vi "温升测试系统.vi"() -> ()   [LabVIEW 2021]
uses:
  <vilib>/Utility/NIReport.llb/Report Type.ctl
  <vilib>/Utility/file.llb/Write Delimited Spreadsheet (string).vi
  <vilib>/Utility/file.llb/Read Delimited Spreadsheet (string).vi
  <userlib>/_MGI/Timing/MGI Wait/MGI Wait (U32).vi
  <vilib>/Waveform/WDTFileIO.llb/Export Waveforms To Spreadsheet File (1D).vi
  <vilib>/Utility/NIReport.llb/Append Text Table to Report (wrap).vi
  <vilib>/Utility/NIReport.llb/NI_report.lvclass
  <vilib>/Utility/NIReport.llb/NI_ReportGenerationCore.lvlib
  <instrlib>/Keithley 27XX/Keithley 27XX.lvlib
  <vilib>/Utility/NIReport.llb/Excel/NI_Excel.lvclass
panel:
  in  "确定按钮 3":bool
  out "当前运行时间":dbl
  out "?":dbl
  in  "样品名称":string
  in  "文本下拉列表":u16(ring) items=["101", "102", "203"]
  out "?":dbl(slide) scale=0.0..200.0
  out "滑动杆":u8(slide) scale=0.0..100.0
  in  "确定按钮 2":bool
  in  "取消按钮":bool
  in  "首选项按钮":bool
  in  "保存按钮":bool
  in  "确定按钮":bool
  in  "停止按钮":bool
  in  "打开按钮":bool
  in  "新建按钮":bool
  in  "?":enum32{"温升曲线", "温升数据", "单曲线显示", "配置面板"}(tab)
  out "?":waveform(dbl)[](graph)
  out "?":i32(listbox)
  out "?":waveform(dbl)(graph)
  out "配置地址":i32(listbox)
  # "工况1"
  # "工况2"
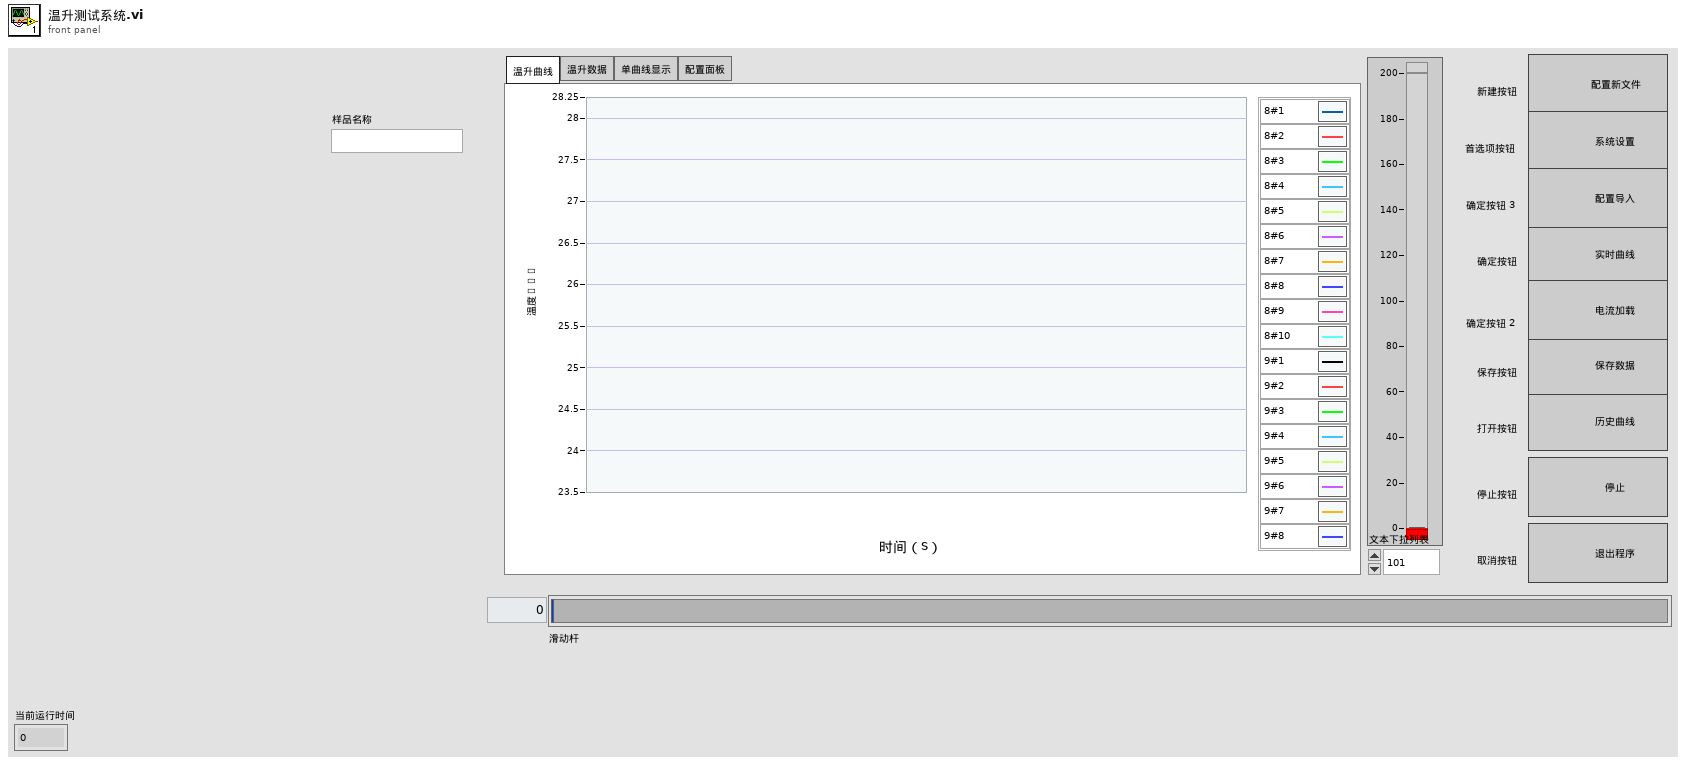
[diagram p1: front panel]
types:
  T1 = enum32{"Invalid", "Standard", "Closed", "Hidden", "Minimized", "Maximized"}
  T2 = cluster{"工况切换地址":refnum<visa-resource-name>, "温度读取":refnum<visa-resource-name>, "电流加载地址":refnum<visa-resource-name>, "RingText.Text":string, "工况1循环次数":dbl, "RingText.Text":string, "工况2循环次数":dbl, "大循环次数":dbl, "测试总时间":dbl, "扫描时间":dbl, "工况模式":enum16{"工况电流", "复合工况"}, "RingText.Text":string, "路径输出":path}
  T3 = typedef "NI_ReportGenerationCore.lvlib/Report Type.ctl" = enum16{"HTML", "Word", "Excel"}
  T4 = cluster{"all rows[0]":string, "all rows[1]":string, "all rows[2]":string, "all rows[3]":string, "all rows[4]":string, "all rows[5]":string, "all rows[6]":string, "all rows[7]":string, "all rows[8]":string, "all rows[9]":string, "all rows[10]":string, "all rows[11]":string, "all rows[12]":string}
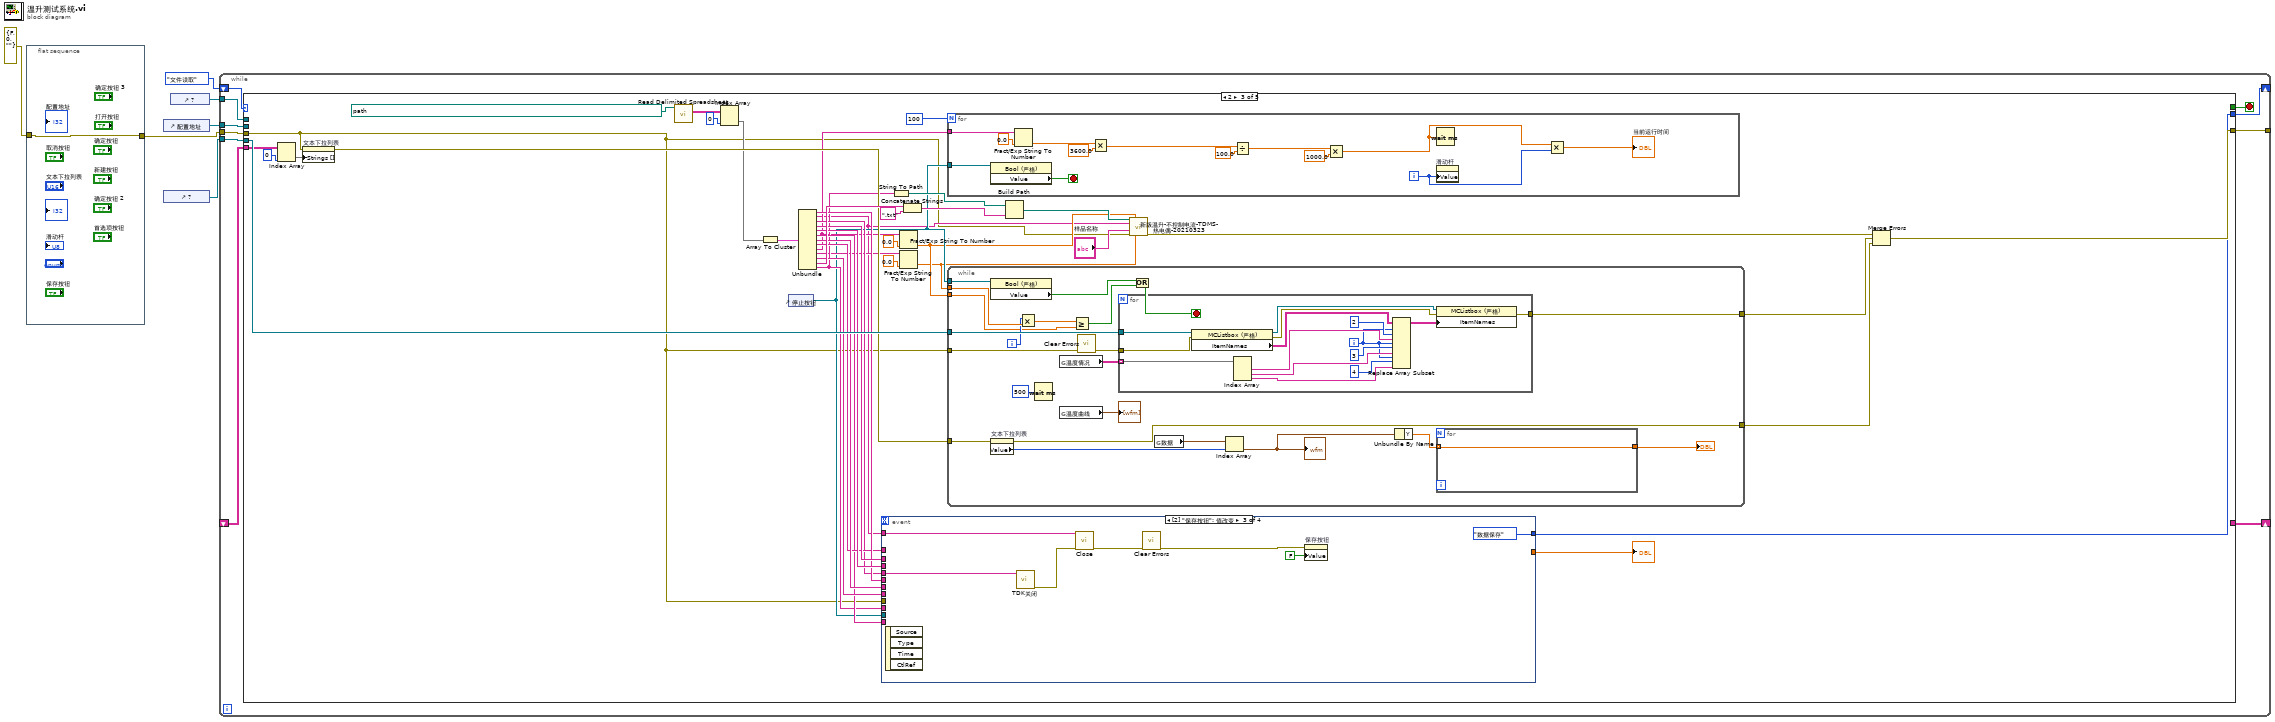
[diagram p0: block diagram]
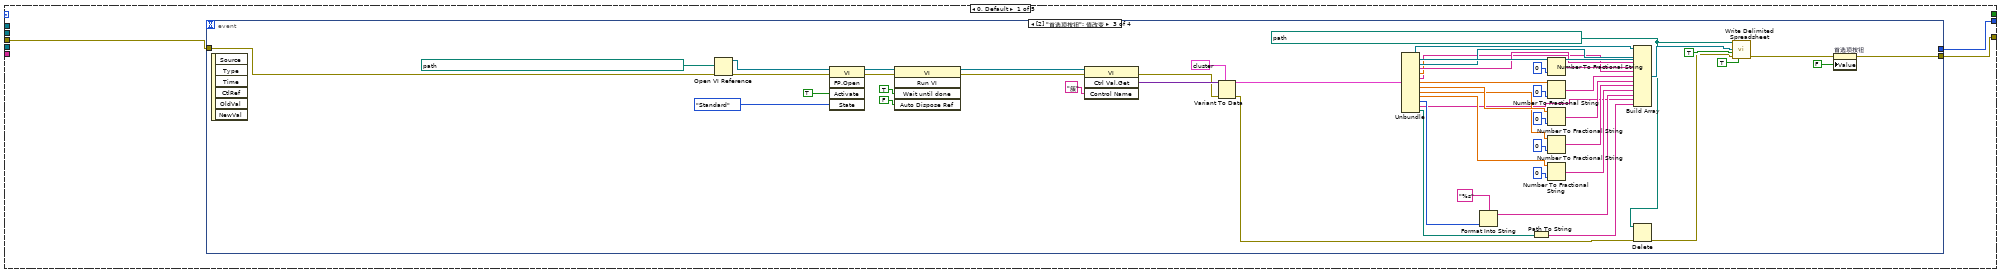
[diagram p2: hidden frame]
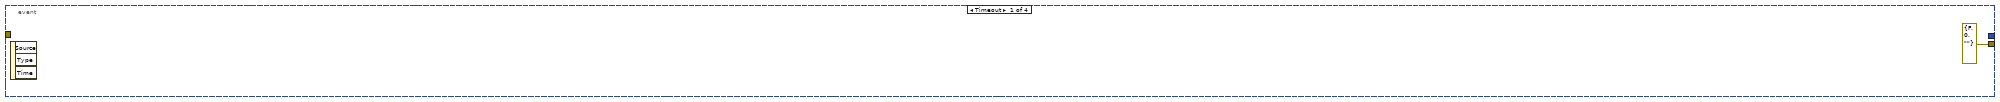
[diagram p3: hidden frame]
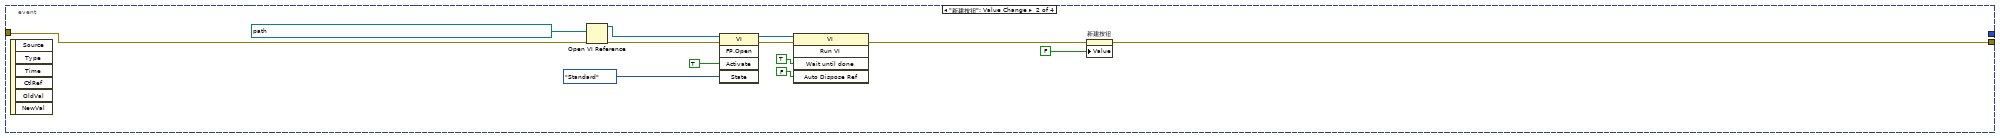
[diagram p4: hidden frame]
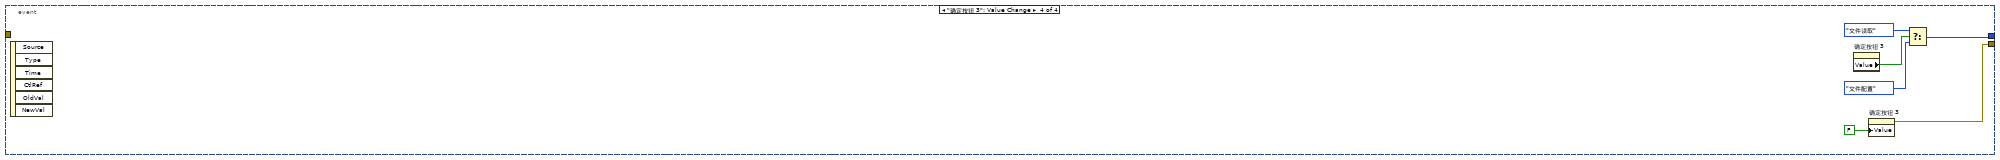
[diagram p5: hidden frame]
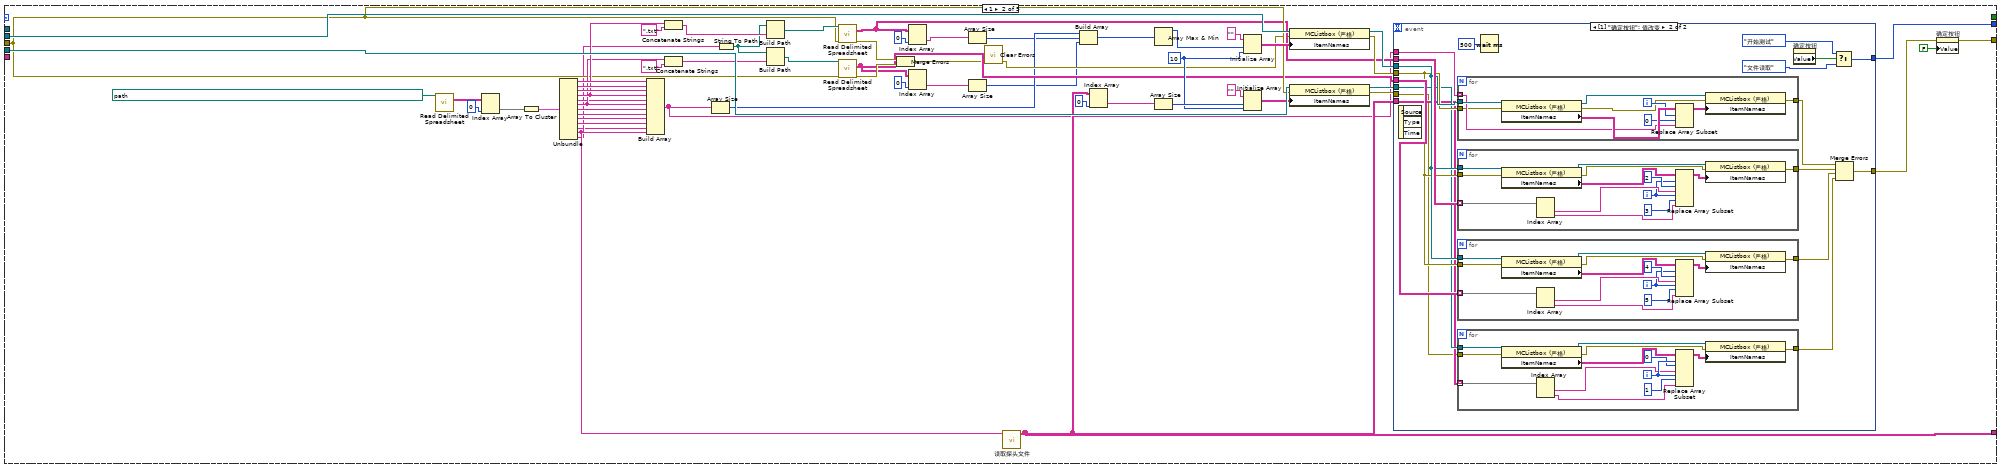
[diagram p6: hidden frame]
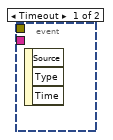
[diagram p7: hidden frame]
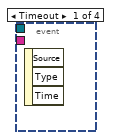
[diagram p8: hidden frame]
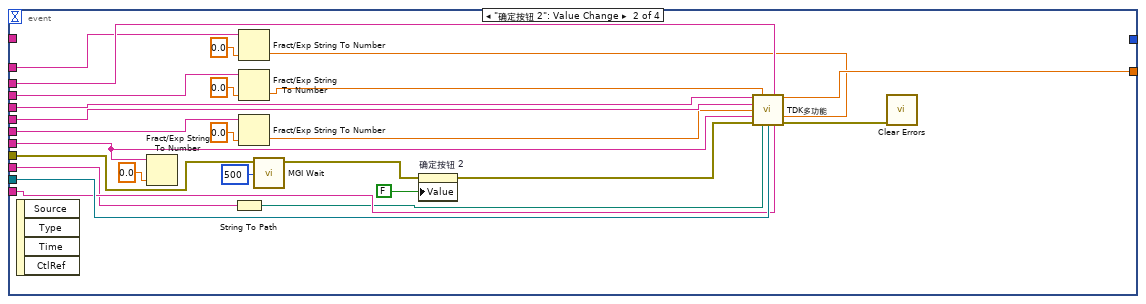
[diagram p9: hidden frame]
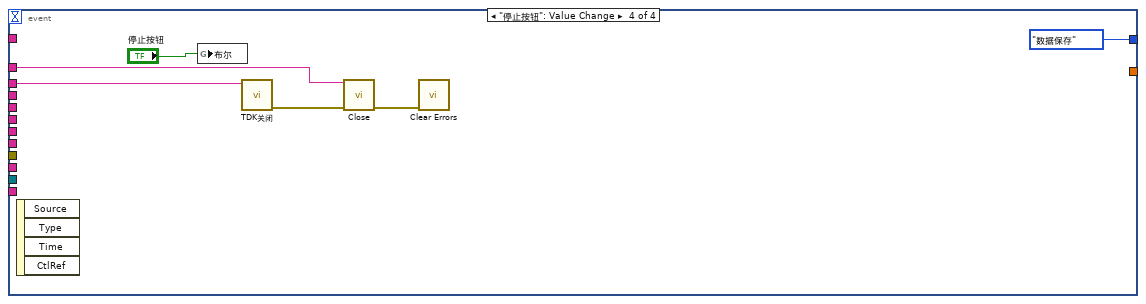
[diagram p10: hidden frame]
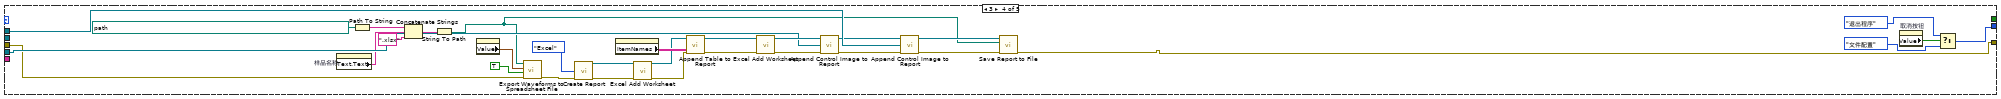
[diagram p11: hidden frame]
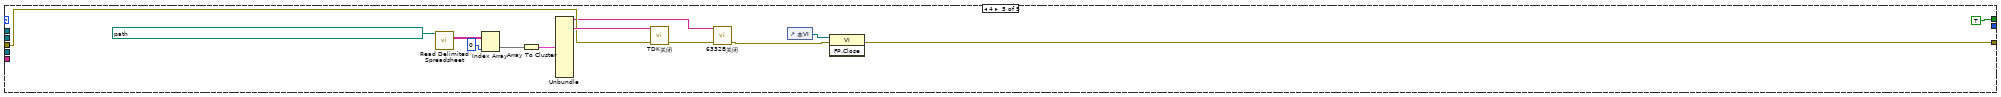
[diagram p12: hidden frame]
diagram:
  n1 = flat-sequence {
    tunnel: [w7] -> w2
    tunnel: errorcluster {"status"=FALSE, "code"=0, "source"=""} ("error in (no error)") -> [w7]
    frame #0 {
    }
  }
  n2 = control-ref of="配置地址"() -> (w5:refnum<vi>)
  n3 = control-ref of="?"() -> (w4:refnum<vi>)
  n4 = control-ref of="?"() -> (w3:refnum<vi>)
  n5 = while {
    tunnel: w5 -> [w17]
    tunnel: w4 -> [w16]
    shift-right: [w15] -> _
    shift-left: enum16{"文件读取", "文件配置", "开始测试", "数据保存", "退出程序"}."文件读取" -> [w8]
    shift-right: [w12] -> _
    shift-left: _ -> [w11]
    tunnel: w3 -> [w10]
    tunnel: w2 -> [w14]
    tunnel: [w13] -> _
    stop <- w9 stop-if-true
    n6 = case shown="2" w8 {
      tunnel: w17 -> [_ w153 _ _ _]
      tunnel: w16 -> [_ w152 w258 w367 _]
      tunnel: [w18 w93 w229 w356 _] -> w15
      tunnel: w14 -> [w19 w126 w223 w363 w393]
      tunnel: [w20 w95 w243 w352 w382] -> w13
      tunnel: [_ w119 _ _ _] -> w12
      tunnel: w11 -> [_ _ w257 _ _]
      tunnel: w10 -> [_ _ _ w366 _]
      tunnel: [_ _ _ _ TRUE] -> w9
      frame 0, Default {
        n7 = event shown="[2] \"首选项按钮\": 值改变" {
          selector: _ -> [_ _ _ _]
          dyn-events: _ -> [_ _ _ _]
          timeout: _ -> [_ _ _ _]
          tunnel: [errorcluster {"status"=FALSE, "code"=0, "source"=""} ("错误输出") w23 w36 w88] -> w20
          tunnel: w19 -> [_ w22 w35 _]
          tunnel: [_ _ _ w89] -> w18
          event Timeout {
            n8 = event-data() -> ()  [unwired: 1 in, 3 out]
          }
          event "新建按钮": Value Change {
            n9 = event-data() -> ()  [unwired: 1 in, 6 out]
            n10 = Open VI Reference(vi path=path "C:/Users/Administrator.CH-202202160008/Desktop/温升测试系统/文件写入.vi" ("VI路径"), error in (no error)=w22) -> (vi reference=w34:refnum<vi>, error out=w30:errorcluster)  [unwired: 4 in]
            n11 = invoke class="VI" method="FP.Open"(reference=w34, error in=w30, "Activate"=TRUE ("激活？"), "State"=T1."Standard" ("状态")) -> (reference out=w33:refnum<vi>, error out=w29:errorcluster)  [unwired: 1 in, 3 out]
            n12 = invoke class="VI" method="Run VI"(reference=w33, error in=w29, "Wait until done"=TRUE ("结束前等待"), "Auto Dispose Ref"=FALSE ("自动销毁引用")) -> (error out=w25:errorcluster)  [unwired: 1 in, 4 out]
            n13 = property on="新建按钮" class="Bool (严格)"(error in=w25, "Value"=FALSE ("新建按钮")) -> (error out=w23:errorcluster)  [unwired: 1 in, 1 out]
          }
          event "首选项按钮": Value Change {
            w37 = path "C:/Users/Administrator.CH-202202160008/Desktop/温升测试系统/仪器配置文件/仪器配置.txt" ("file path (dialog if empty)")
            n14 = event-data() -> ()  [unwired: 1 in, 6 out]
            n15 = Open VI Reference(vi path=path "C:/Users/Administrator.CH-202202160008/Desktop/温升测试系统/系统设置.vi" ("VI路径"), error in (no error)=w35) -> (vi reference=w86:refnum<vi>, error out=w82:errorcluster)  [unwired: 4 in]
            n16 = invoke class="VI" method="FP.Open"(reference=w86, error in=w82, "Activate"=TRUE ("激活？"), "State"=T1."Standard" ("状态")) -> (reference out=w85:refnum<vi>, error out=w81:errorcluster)  [unwired: 1 in, 3 out]
            n17 = invoke class="VI" method="Run VI"(reference=w85, error in=w81, "Wait until done"=TRUE ("结束前等待"), "Auto Dispose Ref"=FALSE ("自动销毁引用")) -> (reference out=w74:refnum<vi>, error out=w73:errorcluster)  [unwired: 1 in, 3 out]
            n18 = invoke class="VI" method="Ctrl Val.Get"(reference=w74, error in=w73, "Control Name"="簇" ("控件名")) -> (error out=w72:errorcluster, "Get Control Value Variant"=w77:variant)  [unwired: 1 in, 2 out]
            n19 = Variant To Data(error in=w72, type=T2 {"工况切换地址"="", "温度读取"="", "电流加载地址"="", "RingText.Text"="新建 文本文档", "工况1循环次数"=1.0, "RingText.Text"="±300", "工况2循环次数"=1.0, "大循环次数"=1.0, "测试总时间"=53.0, "扫描时间"=53.0, "工况模式"=enum."复合工况", "RingText.Text"="", "路径输出"=path "C:/Users/Administrator.CH-202202160008/Desktop/温升测试系统/温升配置文件"} ("簇"), Variant=w77) -> (data=w70:T2, error out=w40:errorcluster)
            n20 = Unbundle(w70) -> ("工况切换地址"=w69:refnum<visa-resource-name>, "温度读取"=w68:refnum<visa-resource-name>, "电流加载地址"=w67:refnum<visa-resource-name>, "RingText.Text"=w66:string, "工况1循环次数"=w65:dbl, "RingText.Text"=w58:string, "工况2循环次数"=w57:dbl, "大循环次数"=w55:dbl, "测试总时间"=w53:dbl, "扫描时间"=w51:dbl, "工况模式"=w49:enum16{"工况电流", "复合工况"}, "RingText.Text"=w46:string, "路径输出"=w45:path)
            n21 = Format Into String(format string="%s" ("格式字符串"), w49) -> (resulting string=w47:string)  [unwired: 2 in, 1 out]
            n22 = Path To String(path=w45) -> (string=w44:string)
            n23 = Number To Fractional String(number=w65, precision (6)=i16 0 ("精度(6)")) -> (F-format string=w64:string)  [unwired: 2 in]
            n24 = Number To Fractional String(number=w57, precision (6)=i16 0 ("精度(6)")) -> (F-format string=w56:string)  [unwired: 2 in]
            n25 = Number To Fractional String(number=w55, precision (6)=i16 0 ("精度(6)")) -> (F-format string=w54:string)  [unwired: 2 in]
            n26 = Number To Fractional String(number=w53, precision (6)=i16 0 ("精度(6)")) -> (F-format string=w52:string)  [unwired: 2 in]
            n27 = Number To Fractional String(number=w51, precision (6)=i16 0 ("精度(6)")) -> (F-format string=w50:string)  [unwired: 2 in]
            n28 = Build Array(w69, w68, w67, w66, w64, w58, w56, w54, w52, w50, w47, w46, w44) -> (w43:refnum<visa-resource-name>[])
            n29 = Delete(path (use dialog)=w37, error in=w40) -> (error out=w39:errorcluster)  [unwired: 3 in, 2 out]
            n30 = call-poly <vilib>:"Write Delimited Spreadsheet.vi"("file path (dialog if empty)"=w37, "1D data"=w43, "append to file? (new file:F)"=TRUE, "error in (no error)"=w39, "transpose? (no:F)"=TRUE) -> ("error out"=w38:errorcluster)  [unwired: 9 in, 1 out]
            n31 = property on="首选项按钮" class="Bool (严格)"(error in=w38, "Value"=FALSE ("首选项按钮")) -> (error out=w36:errorcluster)  [unwired: 1 in, 1 out]
          }
          event "确定按钮 3": Value Change {
            n32 = event-data() -> ()  [unwired: 1 in, 6 out]
            n33 = property on="确定按钮 3" class="Bool (严格)"() -> ("Value"=w92:bool)  [unwired: 2 in, 2 out]
            n34 = property on="确定按钮 3" class="Bool (严格)"("Value"=FALSE ("确定按钮 3")) -> (error out=w88:errorcluster)  [unwired: 2 in, 1 out]
            n35 = Select(t=enum16{"文件配置", "文件读取", "开始测试", "数据保存", "退出程序"}."文件读取", s=w92, f=enum16{"文件配置", "文件读取", "开始测试", "数据保存", "退出程序"}."文件配置") -> (s? t:f=w89:enum16{"文件配置", "文件读取", "开始测试", "数据保存", "退出程序"})
          }
        }
      }
      frame 1 {
        w137 = 10 ("维数大小")
        n36 = call-poly <vilib>:"Read Delimited Spreadsheet.vi"("file path (dialog if empty)"=path "C:/Users/Administrator.CH-202202160008/Desktop/温升测试系统/仪器配置文件/仪器配置.txt") -> ("all rows"=w117:string[][])  [unwired: 9 in, 5 out]
        n37 = Index Array(array=w117, index (col)=0 ("禁用的索引 (列)")) -> (element=w115:string[])  [unwired: 1 in]
        n38 = Array To Cluster(array=w115) -> (cluster=w114:T4)
        n39 = Unbundle(w114) -> ("all rows[0]"=w147:string, "all rows[1]"=w146:string, "all rows[2]"=w145:string, "all rows[3]"=w140:string, "all rows[4]"=w113:string, "all rows[5]"=w132:string, "all rows[6]"=w112:string, "all rows[7]"=w111:string, "all rows[8]"=w110:string, "all rows[9]"=w109:string, "all rows[10]"=w106:string, "all rows[11]"=w144:string, "all rows[12]"=w108:string)
        n40 = Build Array(w147, w146, w145, w140, w113, w132, w112, w111, w110, w109, w106, w144) -> (w103:string[])
        n41 = Concatenate Strings(w140, ".txt" ("字符串")) -> (w141:string)
        n42 = Concatenate Strings(w132, ".txt" ("字符串")) -> (w133:string)
        n43 = Array Size(array=w103) -> (size(s)=w102:i32)
        n44 = String To Path(string=w108) -> (path=w107:path)
        n45 = Build Path(base path=w107, name or relative path=w141) -> (appended path=w143:path)
        n46 = Build Path(base path=w107, name or relative path=w133) -> (appended path=w130:path)
        n47 = call-poly <vilib>:"Read Delimited Spreadsheet.vi"("file path (dialog if empty)"=w143, "error in (no error)"=w126) -> ("all rows"=w122:string[][], "error out"=w128:errorcluster)  [unwired: 8 in, 4 out]
        n48 = call-poly <vilib>:"Read Delimited Spreadsheet.vi"("file path (dialog if empty)"=w130, "error in (no error)"=w126) -> ("all rows"=w124:string[][], "error out"=w127:errorcluster)  [unwired: 8 in, 4 out]
        n49 = Merge Errors(w128, w127) -> (w104:errorcluster)
        n50 = Index Array(array=w122, index (col)=0 ("禁用的索引 (列)")) -> (element=w136:string[])  [unwired: 1 in]
        n51 = Index Array(array=w124, index (col)=0 ("禁用的索引 (列)")) -> (element=w129:string[])  [unwired: 1 in]
        n52 = Array Size(array=w136) -> (size(s)=w101:i32)
        n53 = Array Size(array=w129) -> (size(s)=w100:i32)
        n54 = call <vilib>:"Clear Errors.vi"("error in (no error)"=w104) -> ("error out"=w105:errorcluster)  [unwired: 5 in, 1 out]
        n55 = call "读取探头文件.vi"("字符串"=w144) -> ("all rows"=w119:string[][])  [unwired: 10 in]
        n56 = Build Array(w102, w101, w100) -> (w99:i32[])
        n57 = Index Array(array=w119, index (col)=0 ("禁用的索引 (列)")) -> (element=w148:string[])  [unwired: 1 in]
        n58 = Array Size(array=w148) -> (size(s)=w149:i32)
        n59 = Array Max & Min(array=w99) -> (max value=w98:i32)  [unwired: 3 out]
        n60 = Initialize Array("" ("元素"), w98, w137) -> (w139:string[][])
        n61 = Initialize Array("", w149, w137) -> (w150:string[][])
        n62 = property class="MCListbox (严格)"(reference=w153, error in=w105, "ItemNames"=w139) -> (reference out=w125:refnum<vi>, error out=w123:errorcluster)
        n63 = property class="MCListbox (严格)"(reference=w152, error in=w126, "ItemNames"=w150) -> (reference out=w121:refnum<vi>, error out=w120:errorcluster)
        n64 = event shown="[1] \"确定按钮\": 值改变" {
          selector: _ -> [_ _]
          dyn-events: _ -> [_ _]
          timeout: _ -> [_ _]
          tunnel: w125 -> [_ w165]
          tunnel: w124 -> [_ w167]
          tunnel: w123 -> [_ w163]
          tunnel: w122 -> [_ w166]
          tunnel: w103 -> [_ w164]
          tunnel: w121 -> [_ w162]
          tunnel: w119 -> [_ w161]
          tunnel: w120 -> [_ w160]
          tunnel: [_ w159] -> w96
          tunnel: [_ w154] -> w93
          event Timeout {
            n65 = event-data() -> ()  [unwired: 1 in, 3 out]
          }
          event "确定按钮": Value Change {
            n66 = event-data() -> ()  [unwired: 1 in, 3 out]
            n67 = for {
              tunnel: w165 -> [w207]
              tunnel: w164 -> [w202] mode=indexing
              tunnel: w163 -> [w201]
              tunnel: [w200] -> w168
              i -> [w204]
              n68 = property class="MCListbox (严格)"(reference=w207, error in=w201) -> (reference out=w199:refnum<vi>, error out=w198:errorcluster, "ItemNames"=w206:string[][])
              n69 = Replace Array Subset(array=w206, new element=w202, index (row)=w204, index (col)=0 ("禁用的索引 (列)")) -> (w205:string[][])
              n70 = property class="MCListbox (严格)"(reference=w199, error in=w198, "ItemNames"=w205) -> (error out=w200:errorcluster)  [unwired: 1 out]
            }
            n71 = for {
              tunnel: w165 -> [w197]
              tunnel: w166 -> [w193] mode=indexing
              tunnel: w163 -> [w188]
              tunnel: [w187] -> w169
              i -> [w190]
              n72 = property class="MCListbox (严格)"(reference=w197, error in=w188) -> (reference out=w186:refnum<vi>, error out=w185:errorcluster, "ItemNames"=w196:string[][])
              n73 = Index Array(array=w193) -> (element #1=w192:string, element #2=w191:string)  [unwired: 2 in]
              n74 = Replace Array Subset(array=w196, new element #1=w192, index (row) #1=w190, index (col) #1=2 ("禁用的索引 (列)"), new element #2=w191, index (row) #2=w190, index (col) #2=3 ("禁用的索引 (列)")) -> (w195:string[][])
              n75 = property class="MCListbox (严格)"(reference=w186, error in=w185, "ItemNames"=w195) -> (error out=w187:errorcluster)  [unwired: 1 out]
            }
            n76 = for {
              tunnel: w165 -> [w184]
              tunnel: w167 -> [w176] mode=indexing
              tunnel: w163 -> [w173]
              tunnel: [w172] -> w170
              i -> [w178]
              n77 = property class="MCListbox (严格)"(reference=w184, error in=w173) -> (reference out=w175:refnum<vi>, error out=w174:errorcluster, "ItemNames"=w183:string[][])
              n78 = Index Array(array=w176) -> (element #1=w180:string, element #2=w179:string)  [unwired: 2 in]
              n79 = Replace Array Subset(array=w183, new element #1=w180, index (row) #1=w178, index (col) #1=4 ("禁用的索引 (列)"), new element #2=w179, index (row) #2=w178, index (col) #2=5 ("禁用的索引 (列)")) -> (w182:string[][])
              n80 = property class="MCListbox (严格)"(reference=w175, error in=w174, "ItemNames"=w182) -> (error out=w172:errorcluster)  [unwired: 1 out]
            }
            n81 = for {
              tunnel: w162 -> [w220]
              tunnel: w161 -> [w214] mode=indexing
              tunnel: w160 -> [w209]
              tunnel: [w208] -> w171
              i -> [w217]
              n82 = property class="MCListbox (严格)"(reference=w220, error in=w209) -> (reference out=w211:refnum<vi>, error out=w210:errorcluster, "ItemNames"=w219:string[][])
              n83 = Index Array(array=w214) -> (element #1=w213:string, element #2=w212:string)  [unwired: 2 in]
              n84 = Replace Array Subset(array=w219, new element #1=w213, index (row) #1=w217, index (col) #1=0 ("禁用的索引 (列)"), new element #2=w212, index (row) #2=w217, index (col) #2=1 ("禁用的索引 (列)")) -> (w218:string[][])
              n85 = property class="MCListbox (严格)"(reference=w211, error in=w210, "ItemNames"=w218) -> (error out=w208:errorcluster)  [unwired: 1 out]
            }
            n86 = Wait (ms)(milliseconds to wait=u32 500 ("等待时间（毫秒）")) -> ()  [unwired: 1 out]
            n87 = property on="确定按钮" class="Bool (严格)"() -> ("Value"=w157:bool)  [unwired: 2 in, 2 out]
            n88 = Select(t=enum16{"文件配置", "文件读取", "开始测试", "数据保存", "退出程序"}."开始测试", s=w157, f=enum16{"文件配置", "文件读取", "开始测试", "数据保存", "退出程序"}."文件读取") -> (s? t:f=w154:enum16{"文件配置", "文件读取", "开始测试", "数据保存", "退出程序"})
            n89 = Merge Errors(w168, w169, w170, w171) -> (w159:errorcluster)
          }
        }
        n90 = property on="确定按钮" class="Bool (严格)"(error in=w96, "Value"=FALSE ("确定按钮")) -> (error out=w95:errorcluster)  [unwired: 1 in, 1 out]
      }
      frame 2 {
        n91 = Index Array(array=w257, index (col)=0 ("禁用的索引 (列)")) -> (element=w255:string[])  [unwired: 1 in]
        n92 = property on="文本下拉列表" class="Ring (严格)"(error in=w223, "Strings []"=w255) -> (error out=w246:errorcluster)  [unwired: 1 in, 1 out]
        n93 = call-poly <vilib>:"Read Delimited Spreadsheet.vi"("file path (dialog if empty)"=path "C:/Users/Administrator.CH-202202160008/Desktop/温升测试系统/仪器配置文件/仪器配置.txt") -> ("all rows"=w239:string[][])  [unwired: 9 in, 5 out]
        n94 = Index Array(array=w239, index (col)=0 ("禁用的索引 (列)")) -> (element=w237:string[])  [unwired: 1 in]
        n95 = Array To Cluster(array=w237) -> (cluster=w236:T4)
        n96 = control-ref of="停止按钮"() -> (w228:refnum<vi>)
        n97 = Unbundle(w236) -> ("all rows[0]"=w252:string, "all rows[1]"=w225:string, "all rows[2]"=w241:string, "all rows[3]"=w253:string, "all rows[4]"=w254:string, "all rows[5]"=w248:string, "all rows[6]"=w251:string, "all rows[7]"=w249:string, "all rows[8]"=w231:string, "all rows[9]"=w230:string, "all rows[10]"=w250:string, "all rows[11]"=w260:string, "all rows[12]"=w233:string)
        n98 = event shown="[2] \"保存按钮\": 值改变" {
          selector: _ -> [_ _ _ _]
          dyn-events: _ -> [_ _ _ _]
          timeout: _ -> [_ _ _ _]
          tunnel: w241 -> [_ w337 w344 _]
          tunnel: w254 -> [_ w327 _ _]
          tunnel: w253 -> [_ w336 _ w347]
          tunnel: w252 -> [_ w335 _ _]
          tunnel: w251 -> [_ w325 _ _]
          tunnel: w250 -> [_ w319 _ _]
          tunnel: w249 -> [_ w323 _ w346]
          tunnel: w223 -> [_ w317 _ _]
          tunnel: w233 -> [_ w321 _ _]
          tunnel: w228 -> [_ w334 _ _]
          tunnel: w248 -> [_ w333 _ _]
          tunnel: [_ w332 _ _] -> w247
          tunnel: [_ _ enum16{"文件配置", "文件读取", "开始测试", "数据保存", "退出程序"}."数据保存" enum16{"文件配置", "文件读取", "开始测试", "数据保存", "退出程序"}."数据保存"] -> w229
          tunnel: w225 -> [_ _ w342 _]
          event Timeout {
            n99 = event-data() -> ()  [unwired: 1 in, 3 out]
          }
          event "确定按钮 2": Value Change {
            n100 = event-data() -> ()  [unwired: 1 in, 4 out]
            n101 = Fract/Exp String To Number(string=w319, default (0 dbl)=0.0 ("默认(0 DBL)")) -> ()  [unwired: 2 in, 2 out]
            n102 = String To Path(string=w321) -> (path=w320:path)
            n103 = Fract/Exp String To Number(string=w323, default (0 dbl)=0.0 ("默认(0 DBL)")) -> (number=w322:dbl)  [unwired: 2 in, 1 out]
            n104 = Fract/Exp String To Number(string=w327, default (0 dbl)=0.0 ("默认(0 DBL)")) -> (number=w326:dbl)  [unwired: 2 in, 1 out]
            n105 = Fract/Exp String To Number(string=w325, default (0 dbl)=0.0 ("默认(0 DBL)")) -> (number=w324:dbl)  [unwired: 2 in, 1 out]
            n106 = call-poly <userlib>:"MGI Wait.vi"("ms"=u32 500, "Error In"=w317) -> ("Error Out"=w315:errorcluster)  [unwired: 5 in]
            n107 = property on="确定按钮 2" class="Bool (严格)"(error in=w315, "Value"=FALSE ("确定按钮 2")) -> (error out=w314:errorcluster)  [unwired: 1 in, 1 out]
            n108 = call "TDK多功能.vi"("TDK地址"=w337, "工况1循环次数"=w326, "工况1"=w336, "工况切换地址"=w335, "工况2循环次数"=w324, "字符串"=w319, "大循环次数"=w322, "错误输入（无错误）"=w314, "工况地址"=w320, "Bool引用句柄"=w334, "工况2"=w333) -> ("运行总时间"=w332:dbl, "错误输出"=w313:errorcluster)  [unwired: 3 in]
            n109 = call <vilib>:"Clear Errors.vi"("error in (no error)"=w313) -> ()  [unwired: 5 in, 2 out]
          }
          event "保存按钮": Value Change {
            n110 = event-data() -> ()  [unwired: 1 in, 4 out]
            n111 = call "TDK关闭.vi"("VISA resource name"=w344) -> ("error out"=w341:errorcluster)  [unwired: 10 in]
            n112 = call <instrlib>:"Close.vi"("VISA resource name"=w342, "error in (no error)"=w341) -> ("error out"=w339:errorcluster)  [unwired: 13 in]
            n113 = call <vilib>:"Clear Errors.vi"("error in (no error)"=w339) -> ("error out"=w338:errorcluster)  [unwired: 5 in, 1 out]
            n114 = property on="保存按钮" class="Bool (严格)"(error in=w338, "Value"=FALSE ("保存按钮")) -> ()  [unwired: 1 in, 2 out]
          }
          event "停止按钮": Value Change {
            n115 = event-data() -> ()  [unwired: 1 in, 4 out]
            n116 = global write "数据传输.vi" "布尔"("停止按钮") -> ()
            n117 = call "TDK关闭.vi"("VISA resource name"=w347) -> ("error out"=w350:errorcluster)  [unwired: 10 in]
            n118 = call <instrlib>:"Close.vi"("VISA resource name"=w346, "error in (no error)"=w350) -> ("error out"=w349:errorcluster)  [unwired: 13 in]
            n119 = call <vilib>:"Clear Errors.vi"("error in (no error)"=w349) -> ()  [unwired: 5 in, 2 out]
          }
        }
        "?" <- w247
        n120 = String To Path(string=w233) -> (path=w232:path)
        n121 = Fract/Exp String To Number(string=w231, default (0 dbl)=0.0 ("默认(0 DBL)")) -> (number=w226:dbl)  [unwired: 2 in, 1 out]
        n122 = Fract/Exp String To Number(string=w230, default (0 dbl)=0.0 ("默认(0 DBL)")) -> (number=w222:dbl)  [unwired: 2 in, 1 out]
        n123 = Concatenate Strings(w260, ".txt" ("字符串")) -> (w259:string)
        n124 = for {
          N: 100 -> [_]
          tunnel: w231 -> [w306]
          tunnel: w228 -> [w304]
          i -> [w308]
          stop <- w303 stop-if-true
          n125 = property class="Bool (严格)"(reference=w304) -> ("Value"=w303:bool)  [unwired: 1 in, 2 out]
          n126 = Fract/Exp String To Number(string=w306, default (0 dbl)=0.0 ("默认(0 DBL)")) -> (number=w301:dbl)  [unwired: 2 in, 1 out]
          n127 = Multiply(x=w301, y=3600.0) -> (x*y=w300:dbl)
          n128 = Divide(x=w300, y=100.0) -> (x/y=w310:dbl)
          n129 = Multiply(x=w310, y=1000.0) -> (x*y=w309:dbl)
          n130 = Wait (ms)(milliseconds to wait=w309) -> ()  [unwired: 1 out]
          n131 = property on="滑动杆" class="Slide (严格)"("Value"=w308) -> ()  [unwired: 2 in, 2 out]
          n132 = Multiply(x=w309, y=w308) -> (x*y=→"当前运行时间":dbl)
        }
        n133 = while {
          tunnel: w258 -> [w283]
          tunnel: w246 -> [w282]
          tunnel: [w280] -> w244
          tunnel: w223 -> [w279]
          tunnel: [w281] -> w245
          tunnel: w222 -> [w272]
          tunnel: w226 -> [w269]
          tunnel: w228 -> [w268]
          i -> [w271]
          stop <- w265 stop-if-true
          n134 = property class="Bool (严格)"(reference=w268) -> ("Value"=w267:bool)  [unwired: 1 in, 2 out]
          n135 = property on="文本下拉列表" class="Ring (严格)"(error in=w282) -> (error out=w280:errorcluster, "Value"=w276:u16)  [unwired: 1 in, 1 out]
          n136 = Multiply(x=w271, y=w272) -> (x*y=w270:dbl)
          n137 = Wait (ms)(milliseconds to wait=u32 500 ("等待时间（毫秒）")) -> ()  [unwired: 1 out]
          n138 = global read "数据传输.vi" "温度情况"() -> (w264:string[][])
          n139 = global read "数据传输.vi" "温度曲线"() -> (→"?":waveform(dbl)[])
          n140 = Greater Or Equal?(x=w270, y=w269) -> (x >= y?=w266:bool)
          n141 = call <vilib>:"Clear Errors.vi"("error in (no error)"=w279) -> ("error out"=w278:errorcluster)  [unwired: 5 in, 1 out]
          n142 = for {
            tunnel: w283 -> [w299]
            tunnel: w264 -> [w294] mode=indexing
            tunnel: w278 -> [w289]
            tunnel: [w288] -> w281
            i -> [w287]
            n143 = property class="MCListbox (严格)"(reference=w299, error in=w289) -> (reference out=w291:refnum<vi>, error out=w290:errorcluster, "ItemNames"=w298:string[][])
            n144 = Index Array(array=w294) -> (element #1=w293:string, element #2=w292:string, element #3=w285:string)  [unwired: 3 in]
            n145 = Replace Array Subset(array=w298, new element #1=w293, index (row) #1=w287, index (col) #1=2 ("禁用的索引 (列)"), new element #2=w292, index (row) #2=w287, index (col) #2=3 ("禁用的索引 (列)"), new element #3=w285, index (row) #3=w287, index (col) #3=4 ("禁用的索引 (列)")) -> (w297:string[][])
            n146 = property class="MCListbox (严格)"(reference=w291, error in=w290, "ItemNames"=w297) -> (error out=w288:errorcluster)  [unwired: 1 out]
          }
          n147 = Or(x=w267, y=w266) -> (x .or. y?=w265:bool)
          n148 = global read "数据传输.vi" "数据"() -> (w262:waveform(dbl)[])
          n149 = Index Array(array=w262, index=w276) -> (element=w275:waveform(dbl))
          "?" <- w275
          n150 = Unbundle By Name(w275) -> ("Y"=w274:dbl[])
          n151 = for {
            tunnel: w274 -> [w284] mode=indexing
            tunnel: [w284] -> w273
          }
          "?" <- w273
        }
        n152 = Build Path(base path=w232, name or relative path=w259) -> (appended path=w227:path)
        n153 = call "新版温升-不控制电流-TDMS-热电偶-20210323.vi"("file path (dialog if empty)"=w227, "总记录时间（H）"=w226, "温度读取地址"=w225, "样品名称"="样品名称", "error in (no error)"=w223, "延迟时间（s）"=w222) -> ("错误输出"=w221:errorcluster)  [unwired: 4 in, 5 out]
        n154 = Merge Errors(w221, w245, w244) -> (w243:errorcluster)
      }
      frame 3 {
        n155 = property on="样品名称" class="Str"() -> ("Text.Text"=w362:string)  [unwired: 2 in, 2 out]
        n156 = Path To String(path=path "C:/Users/Administrator.CH-202202160008/Desktop/温升测试系统/实验数据" ("report file path")) -> (string=w359:string)
        n157 = Concatenate Strings(w359, w362, ".xlsx" ("字符串")) -> (w358:string)
        n158 = String To Path(string=w358) -> (path=w357:path)
        n159 = property class="WFChart (严格)"() -> ("Value"=w351:waveform(dbl)[])  [unwired: 2 in, 2 out]
        n160 = call-poly <vilib>:"Export Waveforms to Spreadsheet File.vi"("error in (no error)"=w363, "multiple time columns? (single:F)"=TRUE, "waveforms"=w351, "file path (dialog if empty)"=w357) -> ("error out"=w379:errorcluster)  [unwired: 6 in, 1 out]
        n161 = call <vilib>:"Create Report.vi"("report type"=Report_Type."Excel", "error in (no error)"=w379) -> ("report out"=w371:refnum<class "NI_report.lvclass">, "error out"=w369:errorcluster)  [unwired: 12 in]
        n162 = property class="MCListbox (严格)"() -> ("ItemNames"=w373:string[][])  [unwired: 2 in, 2 out]
        n163 = call <vilib>:"Excel Add Worksheet.vi"("report in"=w371, "error in (no error)"=w369) -> ("report out"=w370:refnum<class "NI_report.lvclass">, "error out"=w368:errorcluster)  [unwired: 12 in]
        n164 = call-poly <vilib>:"Append Table to Report.vi"("report in"=w370, "text data"=w373, "error in (no error)"=w368) -> ("report out"=w374:refnum<class "NI_report.lvclass">, "error out"=w372:errorcluster)  [unwired: 9 in, 2 out]
        n165 = call <vilib>:"Excel Add Worksheet.vi"("report in"=w374, "error in (no error)"=w372) -> ("report out"=w378:refnum<class "NI_report.lvclass">, "error out"=w377:errorcluster)  [unwired: 12 in]
        n166 = call-dynamic "Append Control Image to Report.vi"("report in"=w378, "ctrl reference"=w367, "error in (no error)"=w377) -> ("report out"=w365:refnum<class "NI_report.lvclass">, "error out"=w364:errorcluster)  [unwired: 9 in, 2 out]
        n167 = call-dynamic "Append Control Image to Report.vi"("report in"=w365, "ctrl reference"=w366, "error in (no error)"=w364) -> ("report out"=w376:refnum<class "NI_report.lvclass">, "error out"=w375:errorcluster)  [unwired: 9 in, 2 out]
        n168 = call-dynamic "Save Report to File.vi"("report in"=w376, "report file path"=w357, "error in (no error)"=w375) -> ("error out"=w352:errorcluster)  [unwired: 11 in, 1 out]
        n169 = property on="取消按钮" class="Bool (严格)"() -> ("Value"=w355:bool)  [unwired: 2 in, 2 out]
        n170 = Select(t=enum16{"文件配置", "文件读取", "开始测试", "数据保存", "退出程序"}."退出程序", s=w355, f=enum16{"文件配置", "文件读取", "开始测试", "数据保存", "退出程序"}."文件配置") -> (s? t:f=w356:enum16{"文件配置", "文件读取", "开始测试", "数据保存", "退出程序"})
      }
      frame 4 {
        n171 = call-poly <vilib>:"Read Delimited Spreadsheet.vi"("file path (dialog if empty)"=path "C:/Users/Administrator.CH-202202160008/Desktop/温升测试系统/仪器配置文件/仪器配置.txt") -> ("all rows"=w388:string[][])  [unwired: 9 in, 5 out]
        n172 = Index Array(array=w388, index (col)=0 ("禁用的索引 (列)")) -> (element=w386:string[])  [unwired: 1 in]
        n173 = Array To Cluster(array=w386) -> (cluster=w385:T4)
        n174 = Unbundle(w385) -> ("all rows[0]"=w392:string, "all rows[2]"=w394:string)  [unwired: 11 out]
        n175 = call "TDK关闭.vi"("error in (no error)"=w393, "VISA resource name"=w394) -> ("error out"=w391:errorcluster)  [unwired: 9 in]
        n176 = call "6332B关闭.vi"("错误输入"=w391, "VISA资源名称"=w392) -> ("error out"=w383:errorcluster)  [unwired: 9 in]
        n177 = control-ref of="本VI"() -> (w384:refnum<vi>)
        n178 = invoke class="VI" method="FP.Close"(reference=w384, error in=w383) -> (error out=w382:errorcluster)  [unwired: 1 in, 2 out]
      }
    }
  }
